vi "Main.vi"() -> ()   [LabVIEW 2019, in "MicronTemplateService.lvlib"]
uses:
  MicronTemplateService.lvlib
  Base/Server/Service/ServiceBase.lvclass
  <vilib>/Utility/error.llb/DialogType.ctl
  <vilib>/SLL Toolkit/SLL Queued State Machine/Queue Driver/Create Queue.vi
  <vilib>/SLL Toolkit/SLL Queued State Machine/Queue Driver/Enqueue an Item to Queue.vi
  <vilib>/SLL Toolkit/SLL Queued State Machine/Queue Driver/Dequeue Queue.vi
  <vilib>/SLL Toolkit/SLL Queued State Machine/Queue Driver/Enqueue N Items.vi
  <vilib>/SLL Toolkit/SLL Queued State Machine/Queue Driver/Flush Queue.vi
  <vilib>/SLL Toolkit/SLL Queued State Machine/Queue Driver/Release Queue.vi
  Base/Server/Message/MessageBase.lvclass
  <vilib>/SLL Toolkit/SLL Queued State Machine/SLL QSM.lvlib
  gRPC/Server/Service/GRPCService.lvclass
  <vilib>/SLL Toolkit/SLL String/SLL String.lvlib
panel:
  in  "Stop":bool
  out "Last Message Timestamp":string
  out "Payload":string
  out "Command":string
  in  "Connection String":string="localhost:50051"
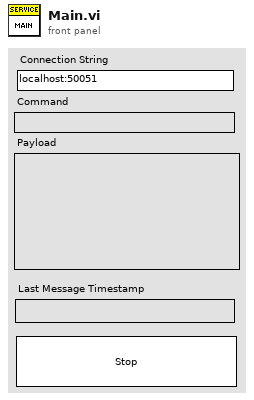
[diagram p1: front panel]
types:
  T1 = cluster{"Flags":cluster{"Source Code?":bool}, "MicronServer":refnum<class "ServiceBase.lvclass">}
  T2 = typedef "MicronServer.lvlib/ServiceBase.lvclass/Micron Args.ctl" = cluster{"Network":string, "Name":string, "Port":i32, "Connection":string, "Args":string[], "Alias":string}
  T3 = typedef "DialogType.ctl" = u16
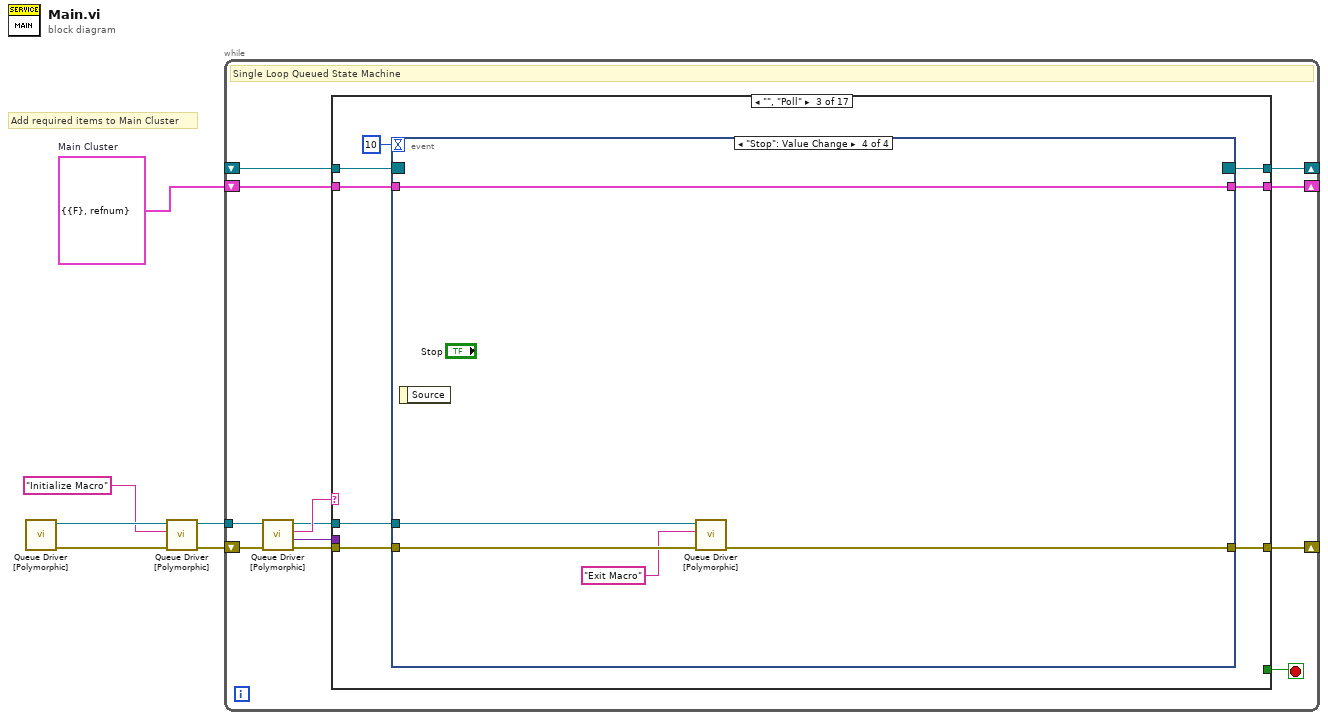
[diagram p0: block diagram]
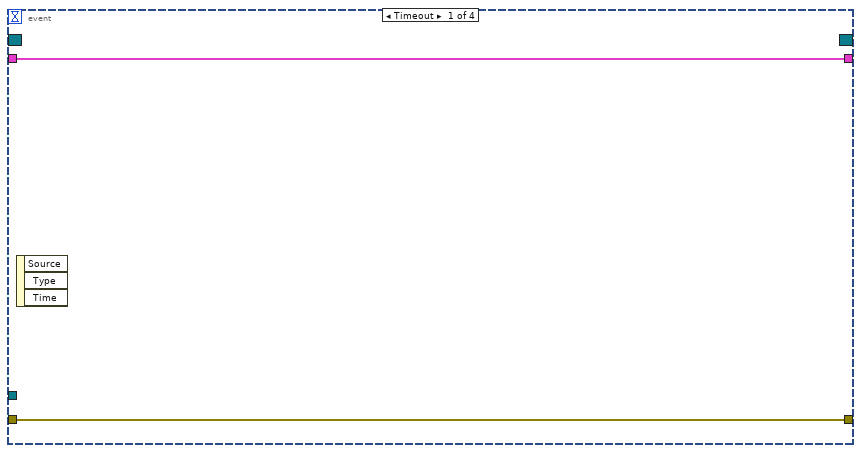
[diagram p4: hidden frame]
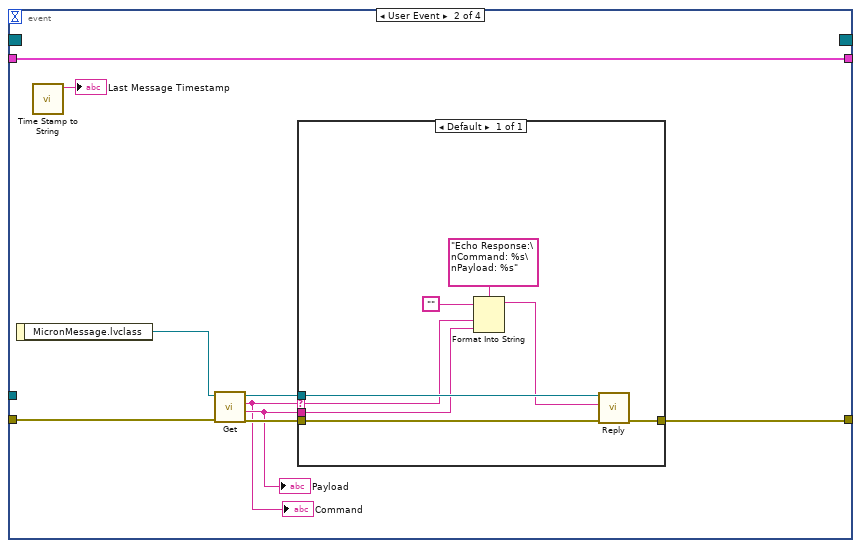
[diagram p5: hidden frame]
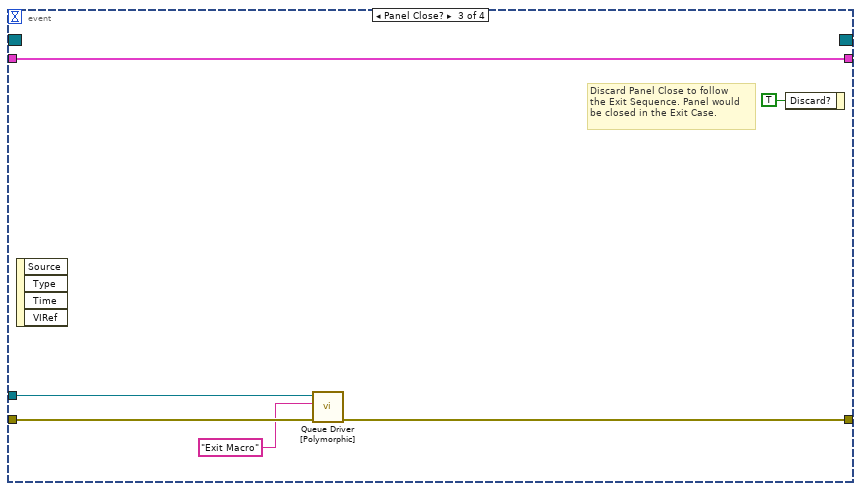
[diagram p6: hidden frame]
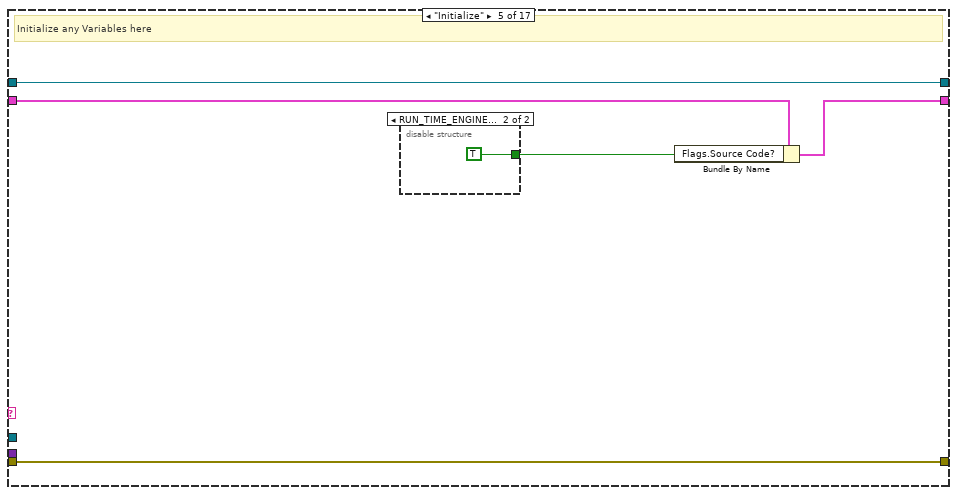
[diagram p8: hidden frame]
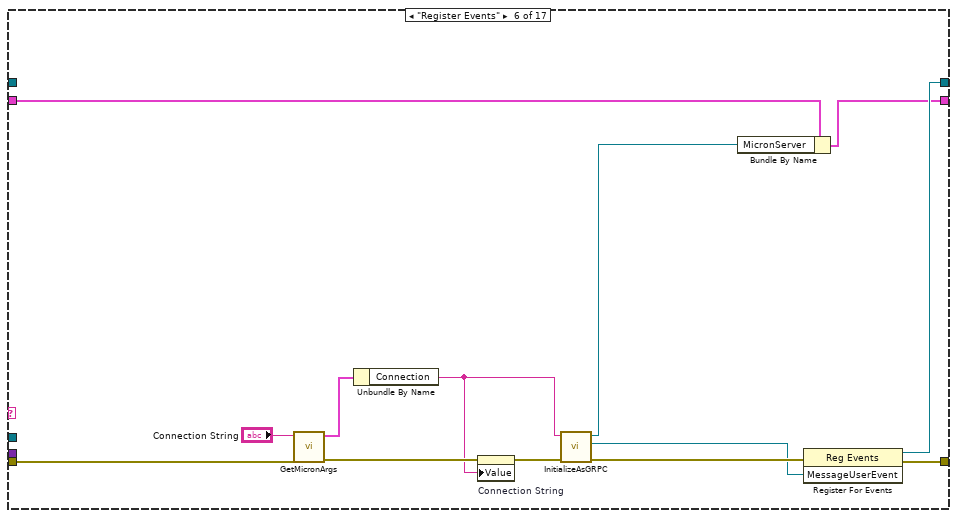
[diagram p10: hidden frame]
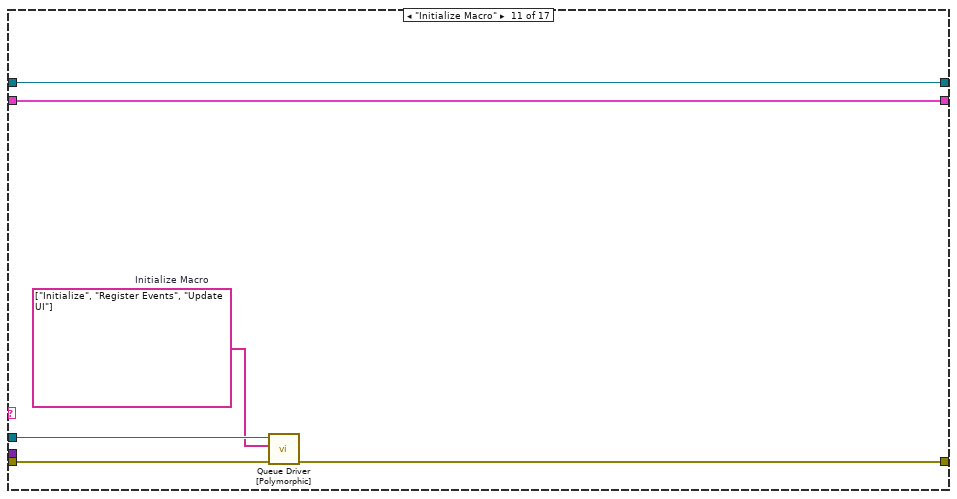
[diagram p15: hidden frame]
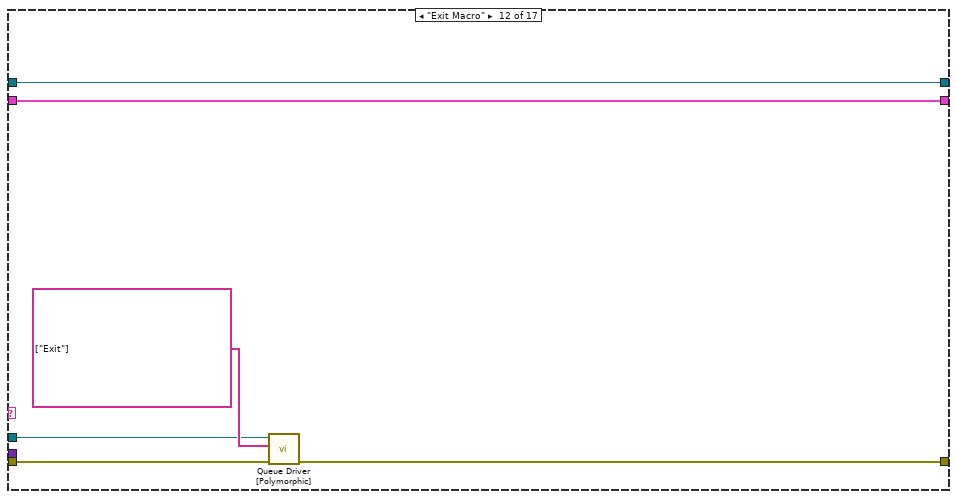
[diagram p16: hidden frame]
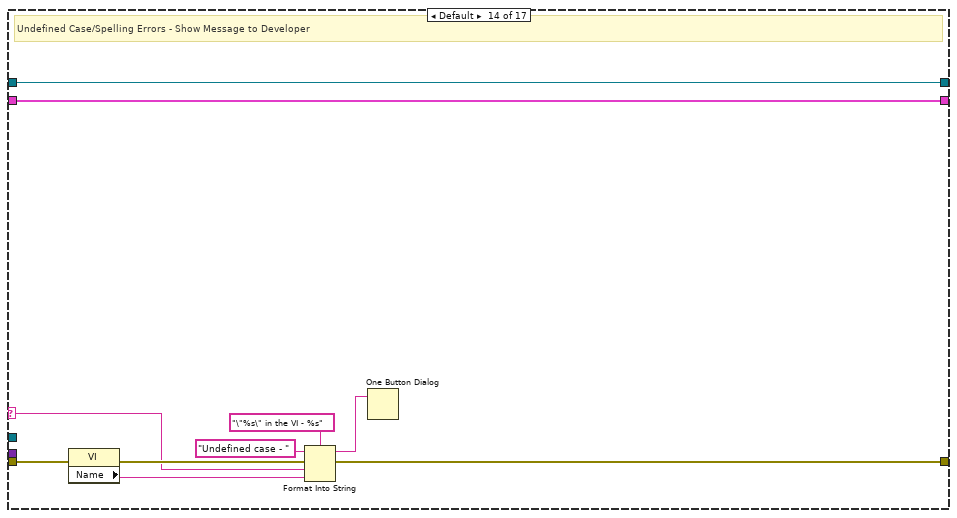
[diagram p18: hidden frame]
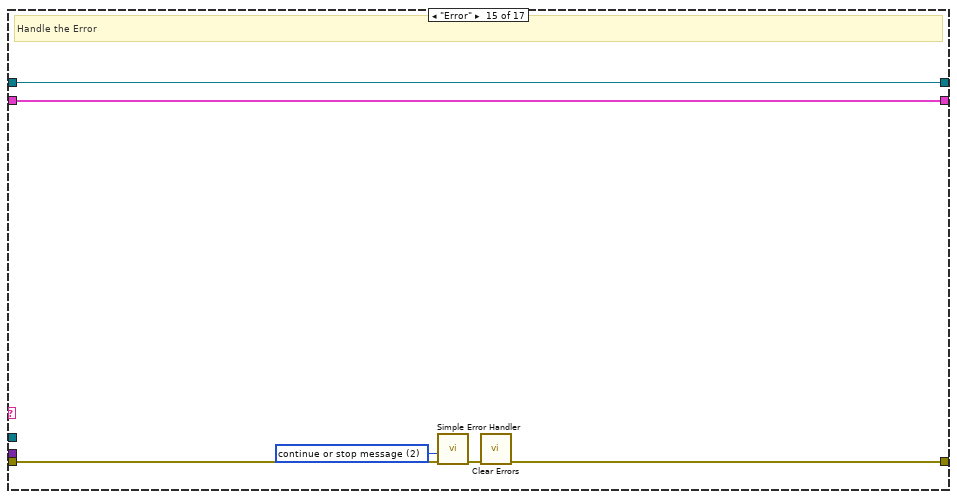
[diagram p19: hidden frame]
diagram:
  w3 = T1 {"Flags"={"Source Code?"=FALSE}, "MicronServer"=refnum}  # Main Cluster
  # "Add required items to Main Cluster"
  n1 = call-poly <vilib>:"Queue Driver [Polymorphic].vi"() -> ("Error Out"=w1:errorcluster, "Queue Ref"=w5:refnum<queue>)  [unwired: 10 in]
  n2 = call-poly <vilib>:"Queue Driver [Polymorphic].vi"("Error In"=w1, "Item to Add"="Initialize Macro", "Queue Ref In"=w5) -> ("Error Out"=w2:errorcluster, "Queue Ref Out"=w6:refnum<queue>)  [unwired: 7 in]
  n3 = while "SLL Queued State Machine" {
    shift-right: [w16] -> _
    shift-left: w2 -> [w18]
    shift-right: [w14] -> _
    shift-left: _ -> [w13]
    shift-right: [w12] -> _
    shift-left: w3 -> [w11]
    tunnel: w6 -> [w9]
    stop <- w15 stop-if-true
    # "Single Loop Queued State Machine"
    n4 = call-poly <vilib>:"Queue Driver [Polymorphic].vi"("Error In"=w18, "Queue Ref In"=w9) -> ("Error Out"=w17:errorcluster, "Data"=w7:variant, "Dequeue"=w10:string, "Queue Ref Out"=w8:refnum<queue>)  [unwired: 6 in]
    n5 = case "QSM Case Structure" shown="\"\", \"Poll\"" w10 {
      selector: w10 -> [_ _ _ _ _ _ _ _ _ _ _ _ _ w112 _ _ _]
      tunnel: w17 -> [w21 w24 w30 w65 w66 w78 w87 w90 w93 w96 w100 w106 w111 w115 w127 w130 w145]
      tunnel: [w21 w24 w31 w65 w66 w84 w87 w90 w93 w96 w99 w105 w111 w118 w125 w130 w141] -> w16
      tunnel: [_ _ _ _ _ _ _ _ _ _ _ _ _ _ _ _ TRUE] -> w15
      tunnel: [w20 w23 w29 w64 w70 w83 w86 w89 w92 w95 w102 w108 w110 w121 w124 w129 w144] -> w14
      tunnel: w13 -> [w20 w23 w28 w64 w70 _ w86 w89 w92 w95 w102 w108 w110 w121 w124 w129 w144]
      tunnel: [w19 w22 w26 w63 w67 w75 w85 w88 w91 w94 w101 w107 w109 w120 w123 w128 w143] -> w12
      tunnel: w11 -> [w19 w22 w27 w63 w68 w82 w85 w88 w91 w94 w101 w107 w109 w120 w123 w128 w143]
      tunnel: w8 -> [_ _ w25 _ _ _ _ _ _ _ w98 w103 _ _ _ _ w134]
      tunnel: w7 -> [_ _ _ _ _ _ _ _ _ _ _ _ _ _ _ _ _]
      frame "/--------------- Read Me -----------------/" {
        # "General Purpose Queue Based State Machine for Any Use Case (main application, module, pop up message etc)\n\nAdvantages:\n1. Lean Project Code Base (dependencies are in vilib).\n2. This template can be safely used in multiple parallel running modules without any issues.\n3. This template can also be safely used even in cases where the VI is configured to be a clone, where multiple \ninstances of the VI could be executing concurrently.\n\nHow to Use:\n1. Add necessary items to the Main Cluster.\n2. Use the Polymorphic Queue Driver for doing any queue operations. \n3. Add any required user events in the \"Register Events\" case. Ignore if not needed.\n4. Use \"Macros\" section for defining any list of state calls, which could be used in multiple places. \nEx: Initialize Macro, might be needed if we need to any reinitialization."
      }
      frame "/------------------ Poll -------------------/" {
      }
      frame "", "Poll" {
        n6 = event shown="[3] \"Stop\": Value Change" {
          selector: w28 -> [_ _ _ _]
          dyn-events: [_ _ _ _] -> w29
          timeout: 10 -> [_ _ _ _]
          tunnel: [w34 w39 w56 w61] -> w31
          tunnel: w30 -> [w34 w40 w57 w62]
          tunnel: w27 -> [w33 w43 w55 w60]
          tunnel: [w33 w43 w55 w60] -> w26
          tunnel: w25 -> [_ _ w53 w59]
          event Timeout {
            n7 = event-data() -> ()  [unwired: 1 in, 3 out]
          }
          event User Event {
            n8 = event-data() -> ("MicronMessage.lvclass"=w38:refnum<class "MessageBase.lvclass">)  [unwired: 1 in]
            n9 = call <vilib>:"Time Stamp to String.vi"() -> ("Output String"=→"Last Message Timestamp":string)  [unwired: 11 in]
            n10 = call-dynamic "Get.vi"("error in (no error)"=w40, "MicronMessage in"=w38) -> ("error out"=w42:errorcluster, "Payload"=w36:string, "Command"=w35:string, "MicronMessage out"=w41:refnum<class "MessageBase.lvclass">)  [unwired: 6 in]
            "Payload" <- w36
            "Command" <- w35
            n11 = case shown="Default" w35 {
              selector: w35 -> [w44]
              tunnel: w42 -> [w51]
              tunnel: w41 -> [w50]
              tunnel: [w46] -> w39
              tunnel: w36 -> [w45]
              frame Default {
                n12 = Format Into String(format string="Echo Response:\nCommand: %s\nPayload: %s", initial string="", w44, w45) -> (resulting string=w47:string)  [unwired: 1 in, 1 out]
                n13 = call-dynamic "Reply.vi"("error in (no error)"=w51, "Response"=w47, "MicronMessage in"=w50) -> ("error out"=w46:errorcluster)  [unwired: 7 in, 1 out]
              }
            }
          }
          event Panel Close? {
            # "Discard Panel Close to follow\nthe Exit Sequence. Panel would\nbe closed in the Exit Case."
            n14 = event-data() -> ()  [unwired: 1 in, 4 out]
            n15 = call-poly <vilib>:"Queue Driver [Polymorphic].vi"("Error In"=w57, "Item to Add"="Exit Macro" ("Enqueue"), "Queue Ref In"=w53) -> ("Error Out"=w56:errorcluster)  [unwired: 7 in, 1 out]
            n16 = event-data("Discard?"=TRUE) -> ()  [unwired: 1 in, 1 out]
          }
          event "Stop": Value Change {
            n17 = event-data() -> ()  [unwired: 1 in, 1 out]
            n18 = call-poly <vilib>:"Queue Driver [Polymorphic].vi"("Error In"=w62, "Item to Add"="Exit Macro" ("Enqueue"), "Queue Ref In"=w59) -> ("Error Out"=w61:errorcluster)  [unwired: 7 in, 1 out]
          }
        }
      }
      frame "/--------------- Initialize -----------------/" {
      }
      frame "Initialize" {
        # "Initialize any Variables here"
        n19 = disable-structure shown="RUN_TIME_ENGINE==False" {
          disable-tunnel: [_ TRUE] -> w69
          frame condition #0 {
          }
          frame condition #1 (active) {
          }
        }
        n20 = Bundle By Name(cluster=w68, "Flags.Source Code?"=w69) -> (w67:T1)
      }
      frame "Register Events" {
        n21 = call "GetMicronArgs.vi"("error in (no error)"=w78, "Default Connection String"="Connection String") -> ("error out"=w80:errorcluster, "Micron Args"=w81:T2)  [unwired: 8 in]
        n22 = Unbundle By Name(w81) -> ("Connection"=w73:string)
        n23 = property on="Connection String" class="Str"(error in=w80, "Value"=w73) -> (error out=w79:errorcluster)  [unwired: 1 in, 1 out]
        n24 = call "InitializeAsGRPC.vi"("error in (no error)"=w79, "Connection String"=w73) -> ("error out"=w77:errorcluster, "MessageUserEvent"=w76:refnum<user-event>, "MicronServer"=w74:refnum<class "ServiceBase.lvclass">)  [unwired: 7 in]
        n25 = Bundle By Name(cluster=w82, "MicronServer"=w74) -> (w75:T1)
        n26 = register-events(error in=w77, w76) -> (reference out=w83:refnum<event-registration>, error out=w84:errorcluster)  [unwired: 1 in]
      }
      frame "/---------- Custom Case Splitter ----------/" {
      }
      frame "/-------------- User Interface --------------/" {
        # "Duplicate this case to create additional case splitters for readability"
      }
      frame "Update UI" {
        # "Update Front Panel Controls in this Case"
      }
      frame "/----------------- Macros -----------------/" {
      }
      frame "Initialize Macro" {
        w97 = string[] ["Initialize", "Register Events", "Update UI"]  # Initialize Macro
        n27 = call-poly <vilib>:"Queue Driver [Polymorphic].vi"("Error In"=w100, "Enqueue N"=w97, "Queue Ref In"=w98) -> ("Error Out"=w99:errorcluster)  [unwired: 7 in, 1 out]
      }
      frame "Exit Macro" {
        n28 = call-poly <vilib>:"Queue Driver [Polymorphic].vi"("Error In"=w106, "Enqueue N"=string[] ["Exit"], "Queue Ref In"=w103) -> ("Error Out"=w105:errorcluster)  [unwired: 7 in, 1 out]
      }
      frame "/-------------- Error Handler--------------/" {
      }
      frame Default {
        # "Undefined Case/Spelling Errors - Show Message to Developer"
        n29 = property class="VI"(error in=w115) -> (error out=w114:errorcluster, "Name"=w113:string)  [unwired: 1 in, 1 out]
        n30 = Format Into String(format string="\"%s\" in the VI - %s" ("message"), initial string="Undefined case - ", error in=w114, w112, w113) -> (resulting string=w116:string, error out=w118:errorcluster)
        n31 = One Button Dialog(message=w116) -> ()  [unwired: 1 in, 1 out]
      }
      frame "Error" {
        w122 = T3 2 items=["no dialog", "OK message", "continue or stop message", "OK message + warnings", "continue/stop + warnings"] ("type of dialog (OK msg:1)")
        # "Handle the Error"
        n32 = call <vilib>:"Simple Error Handler.vi"("type of dialog (OK msg:1)"=w122, "error in (no error)"=w127) -> ("error out"=w126:errorcluster)  [unwired: 3 in, 4 out]
        n33 = call <vilib>:"Clear Errors.vi"("error in (no error)"=w126) -> ("error out"=w125:errorcluster)  [unwired: 5 in, 1 out]
      }
      frame "/------------------- Exit --------------------/" {
      }
      frame "Exit" {
        n34 = call-poly <vilib>:"Queue Driver [Polymorphic].vi"("Error In"=w145, "Queue Ref In"=w134) -> ("Error Out"=w146:errorcluster, "Queue Ref Out"=w133:refnum<queue>)  [unwired: 7 in, 1 out]
        n35 = Unbundle By Name(w143) -> ("Flags.Source Code?"=w136:bool, "MicronServer"=w131:refnum<class "ServiceBase.lvclass">)
        n36 = call-poly <vilib>:"Queue Driver [Polymorphic].vi"("Error In"=w146, "Queue Ref In"=w133) -> ("Error Out"=w142:errorcluster)  [unwired: 9 in]
        n37 = call-dynamic "CloseCore.vi"("error in (no error)"=w142, "MicronServer in"=w131) -> ("error out"=w132:errorcluster)  [unwired: 8 in, 1 out]
        n38 = Call Chain() -> (call chain=w140:string[])
        n39 = Array Size(array=w140) -> (size(s)=w139:i32)
        n40 = Equal?(x=w139, y=1) -> (x = y?=w137:bool)
        n41 = And(x=w136, y=w137) -> (x .and. y?=w135:bool)
        n42 = case "Skip Panel Close when in Source\nCode and is the top most caller" shown="False" w135 {
          tunnel: w132 -> [w149 w151]
          tunnel: [w150 w151] -> w141
          frame False {
            # "Close Panel"
            n43 = invoke class="VI" method="FP.Close"() -> (error out=w148:errorcluster)  [unwired: 3 in, 2 out]
            n44 = Merge Errors(w149, w148) -> (w150:errorcluster)
          }
          frame True {
            # "Do Not Close Panel"
          }
        }
      }
    }
  }
